vi "Start Live Mode.vi"(8 "error in (no error)":errorcluster, 11 "Orca-Flash 4.0 V2 in":refnum<class "Orca-Flash 4.0 V2.lvclass">) -> (0 "error out":errorcluster, 3 "Orca-Flash 4.0 V2 out":refnum<class "Orca-Flash 4.0 V2.lvclass">)   [LabVIEW 2015]
uses:
  Orca-Flash 4.0 V2.lvclass
  Resources/Type Defs/Flash Settings.ctl
panel:
  in  "Camera Settings":T1={"Exposure Time"=0.1, "Binning"=enum."2x2", "Scan Mode (Flash)"=enum."Fast", "Trigger Mode (Flash)"=enum."Fast", "Frames to Acquire"=1000.0} {"Exposure Time" min=0.001 max=10.0 step=0.001}
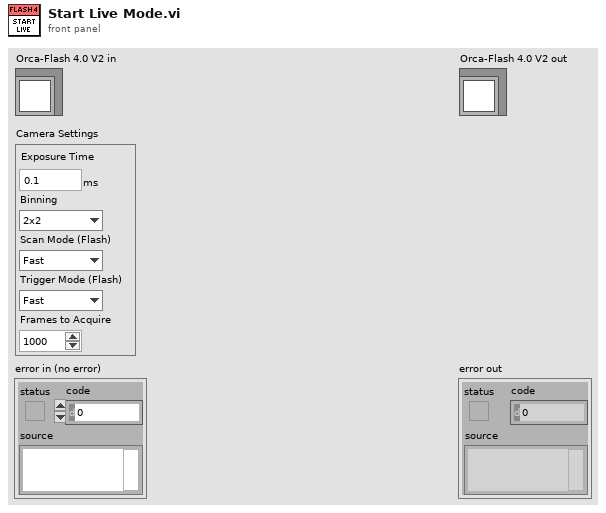
[diagram p1: front panel]
types:
  T1 = typedef "Flash Settings.ctl" = cluster{"Exposure Time":dbl[unit], "Binning":enum16{"1x1", "2x2", "4x4"}, "Scan Mode (Flash)":enum16{"Fast", "Slow"}, "Trigger Mode (Flash)":enum16{"Fast", "Standard"}, "Frames to Acquire":dbl}
  T2 = cluster{"height":u32, "width":u32, "datatype":u32}
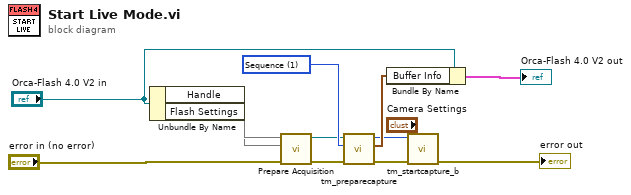
[diagram p0: block diagram]
diagram:
  w5 = 1 items=["Snap", "Sequence"] ("Capture mode")
  n1 = Unbundle By Name("Orca-Flash 4.0 V2 in") -> ("Handle"=w4, "Flash Settings"=w1)
  n2 = call "Prepare Acquisition.vi"("error in (no error)"="error in (no error)", "Flash Settings"=w1, "Orca-Flash 4.0 in"=w4) -> ("error out"=w2:errorcluster, "Orca-Flash 4.0 out"=w3:refnum<class "Orca-Flash 4.0 V2.lvclass">)  [unwired: 7 in]
  n3 = call <userlib>:"tm_preparecapture.vi"("error in (no error)"=w2, "Capture mode"=w5, "Handle in"=w3) -> ("error out"=w6:errorcluster, "Buffer Info"=w8:T2, "Handle out"=w7:u32)  [unwired: 5 in, 1 out]
  n4 = Bundle By Name(cluster="Orca-Flash 4.0 V2 in", "Buffer Info"=w8) -> (→"Orca-Flash 4.0 V2 out":cluster{})
  n5 = call <userlib>:"tm_startcapture_b.vi"("error in (no error)"=w6, "Handle in"=w7) -> ("error out"=→"error out":errorcluster)  [unwired: 8 in, 1 out]
